vi "Software Update HCC Get Latest Data Folder.vi"(8 "Error In":errorcluster, 10 "New Software Location":path, 11 "Path Build List Sub Input":path) -> (0 "Error Out":errorcluster, 3 "Path Build List Sub Output":path)   [LabVIEW 2016]
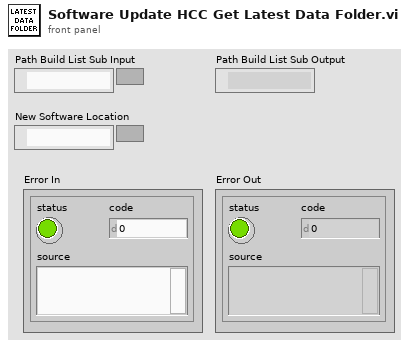
[diagram p1: front panel]
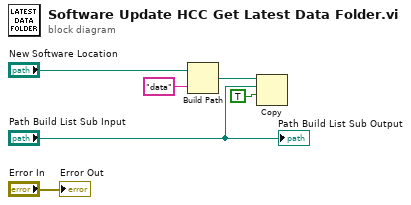
[diagram p0: block diagram]
diagram:
  n1 = Build Path(base path="New Software Location", name or relative path="data") -> (appended path=w3:path)
  n2 = Copy(9:TRUE ("overwrite (F)"), 10:"Path Build List Sub Input", 11:w3) -> ()  [unwired: 2 in, 3 out]
  "Error Out" <- "Error In"
  "Path Build List Sub Output" <- "Path Build List Sub Input"
